vi "SettingUp.vi"(8 "ErrorQueue":refnum<queue>, 9 "PreSetup":refnum<queue>, 10 "VIRef":refnum<vi>, 11 "Actor":refnum<class "Actor.lvclass">) -> (2 "EventRegistrationRef":refnum<event-registration>, 3 "Actor":refnum<class "Actor.lvclass">, 4 "Error":errorcluster)   [LabVIEW 2020, in "jettl.lvlib"]
uses:
  jettl.lvlib
  Lifetime.ctl
  Actor/Actor.lvclass
  PreSetup.ctl
  Message.ctl
  Message/Message.lvclass
panel:
  out "ContinueToRunning":bool
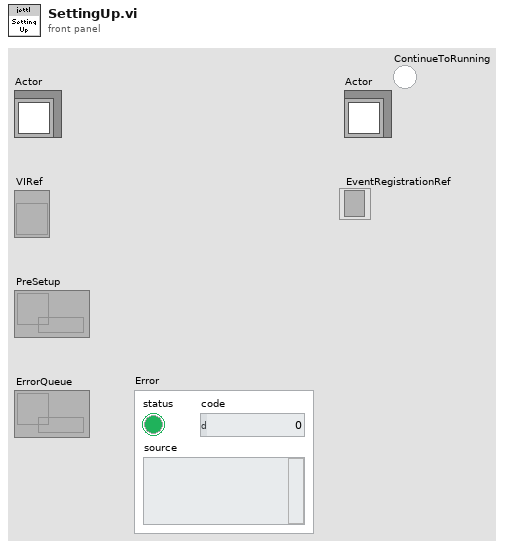
[diagram p1: front panel]
types:
  T1 = typedef "jettl.lvlib/PreSetup.ctl" = cluster{"VIRef":refnum<vi>, "ContinueToRunning":refnum<queue>}
  T2 = typedef "jettl.lvlib/Lifetime.ctl" = enum16{"Setup", "TeardownBeforeStart", "Start", "Running", "Stop", "TeardownAfterStart"}
  T3 = typedef "jettl.lvlib/Base.ctl" = cluster{"Lifetime":T2, "SelfActor":T4, "MediatorActor":T4, "ComponentActorMap":T9}
  T4 = typedef "jettl.lvlib/Actor.ctl" = cluster{"Messages":T5, "ActorAlias":string, "ActorType":T8, "Transport":refnum<user-event>, "EventRegistrationRef":refnum<event-registration>, "VIRef":refnum<vi>}
  T5 = typedef "jettl.lvlib/Messages.ctl" = cluster{"Listen":T6, "TellSelf":T6, "TellMediator":T6, "TellComponentMap":T7}
  T6 = typedef "jettl.lvlib/MessageSet.ctl" = set{refnum<class "Message.lvclass">}
  T7 = typedef "jettl.lvlib/TellComponentMap.ctl" = map{string, T6}
  T8 = typedef "jettl.lvlib/ActorType.ctl" = enum16{"Mediator", "Component"}
  T9 = typedef "jettl.lvlib/ComponentActorMap.ctl" = map{string, T4}
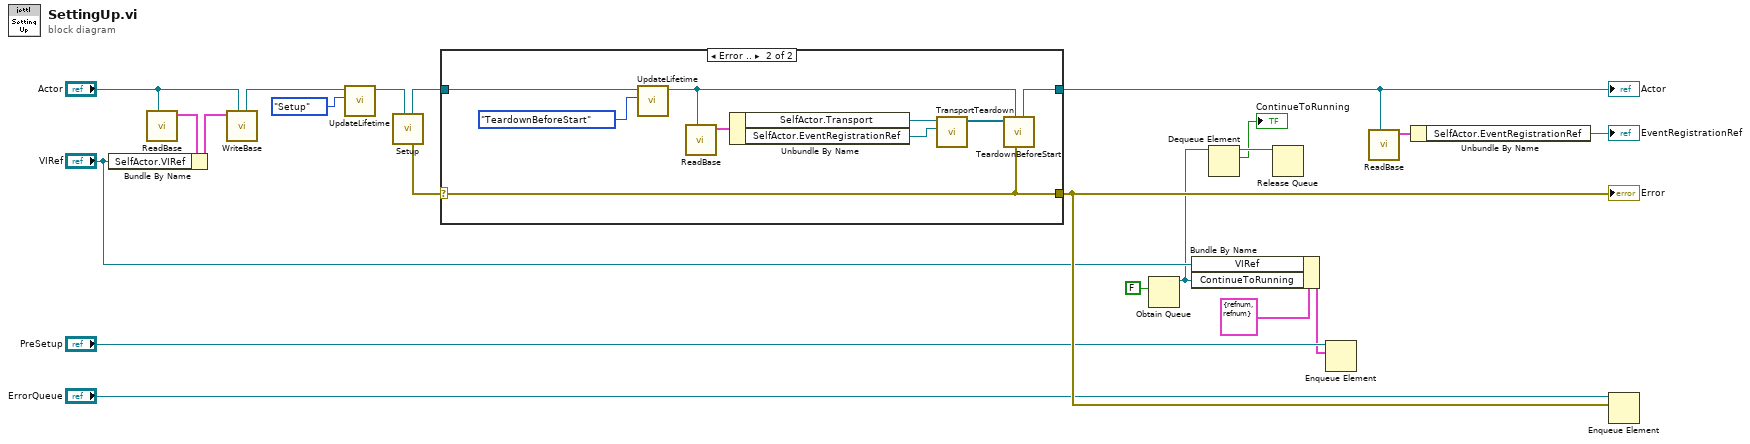
[diagram p0: block diagram]
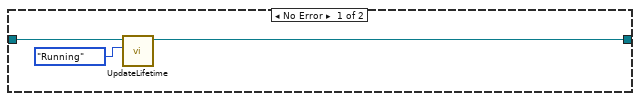
[diagram p2: hidden frame]
diagram:
  n1 = call-dynamic "ReadBase.vi"("Actor"="Actor") -> ("Base"=w20:T3)  [unwired: 10 in]
  n2 = Bundle By Name(cluster=w20, "SelfActor.VIRef"="VIRef") -> (w19:T3)
  n3 = call-dynamic "WriteBase.vi"("Actor"="Actor", "Base"=w19) -> ("Actor"=w13:refnum<class "Actor.lvclass">)  [unwired: 9 in]
  n4 = call "UpdateLifetime.vi"("Lifetime"=Lifetime."Setup", "Actor"=w13) -> ("Actor"=w14:refnum<class "Actor.lvclass">)  [unwired: 9 in]
  n5 = call-dynamic "Setup.vi"("Actor"=w14) -> ("Error"=w17:errorcluster, "Actor"=w18:refnum<class "Actor.lvclass">)  [unwired: 9 in]
  n6 = case shown="Error .." w17 {
    selector: w17 -> [_ w29]
    tunnel: w18 -> [w22 w27]
    tunnel: [_ w29] -> w21
    tunnel: [w23 w32] -> w12
    frame No Error {
      n7 = call "UpdateLifetime.vi"("Lifetime"=Lifetime."Running", "Actor"=w22) -> ("Actor"=w23:refnum<class "Actor.lvclass">)  [unwired: 9 in]
    }
    frame Error {
      n8 = call "UpdateLifetime.vi"("Lifetime"=Lifetime."TeardownBeforeStart", "Actor"=w27) -> ("Actor"=w28:refnum<class "Actor.lvclass">)  [unwired: 9 in]
      n9 = call-dynamic "ReadBase.vi"("Actor"=w28) -> ("Base"=w33:T3)  [unwired: 10 in]
      n10 = Unbundle By Name(w33) -> ("SelfActor.Transport"=w31:refnum<user-event>, "SelfActor.EventRegistrationRef"=w26:refnum<event-registration>)
      n11 = call "TransportTeardown.vi"("EventRegistrationRef"=w26, "Transport"=w31) -> ("UnheardMessages"=w30:refnum<class "Message.lvclass">[])  [unwired: 9 in]
      n12 = call-dynamic "TeardownBeforeStart.vi"("Error"=w29, "Actor"=w28, "UnheardMessages"=w30) -> ("Actor"=w32:refnum<class "Actor.lvclass">)  [unwired: 8 in]
    }
  }
  "Actor" <- w12
  "Error" <- w21
  n13 = Obtain Queue(element data type=FALSE) -> (queue out=w3:refnum<queue>)  [unwired: 4 in, 2 out]
  n14 = Bundle By Name(cluster=T1 {"VIRef"=refnum, "ContinueToRunning"=refnum} ("element"), "VIRef"="VIRef", "ContinueToRunning"=w3) -> (w7:T1)
  n15 = Dequeue Element(queue=w3) -> (queue out=w2:refnum<queue>, element=→"ContinueToRunning":bool)  [unwired: 2 in, 2 out]
  n16 = Release Queue(queue=w2) -> ()  [unwired: 2 in, 3 out]
  n17 = Enqueue Element(queue="PreSetup", element=w7) -> ()  [unwired: 2 in, 3 out]
  n18 = call-dynamic "ReadBase.vi"("Actor"=w12) -> ("Base"=w11:T3)  [unwired: 10 in]
  n19 = Unbundle By Name(w11) -> ("SelfActor.EventRegistrationRef"=→"EventRegistrationRef":refnum<event-registration>)
  n20 = Enqueue Element(queue="ErrorQueue", element=w21) -> ()  [unwired: 2 in, 3 out]
